vi "ISMBUS_DecodeModuleProtocol.vi"(8 "Fehler (Eingang - kein Fehler)":errorcluster, 11 "ModuleProtocolIndex":i32) -> (0 "error (Ausgang)":errorcluster caption="Fehler  (Ausgang)", 3 "ModuleProtocolString":string)   [LabVIEW 2016]
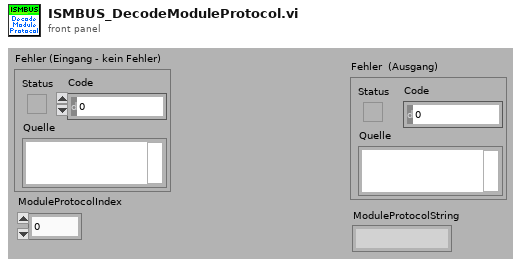
[diagram p1: front panel]
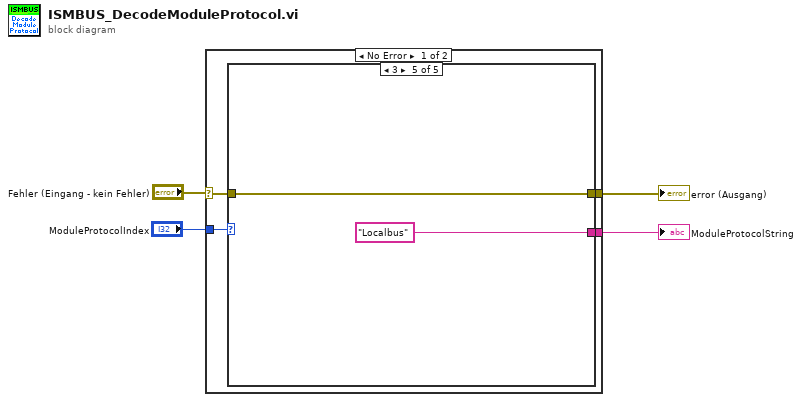
[diagram p0: block diagram]
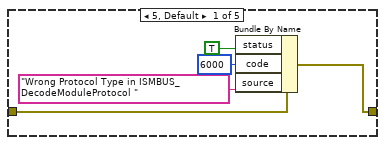
[diagram p2: hidden frame]
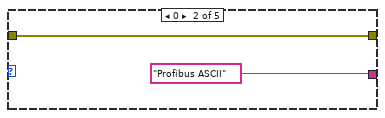
[diagram p3: hidden frame]
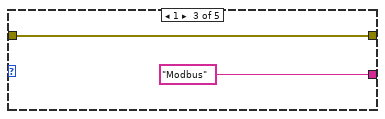
[diagram p4: hidden frame]
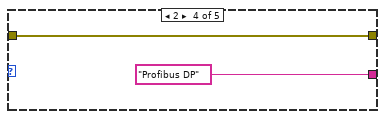
[diagram p5: hidden frame]
diagram:
  n1 = case shown="No Error" "Fehler (Eingang - kein Fehler)" {
    selector: "Fehler (Eingang - kein Fehler)" -> [w6 w22]
    tunnel: "ModuleProtocolIndex" -> [w8 _]
    tunnel: [w7 _] -> w1
    tunnel: [w5 w22] -> w2
    frame No Error {
      n2 = case shown="3" w8 {
        tunnel: [_ "Profibus ASCII" "Modbus" "Profibus DP" "Localbus"] -> w7
        tunnel: w6 -> [w12 w15 w16 w18 w20]
        tunnel: [w13 w15 w16 w18 w20] -> w5
        frame 5, Default {
          n3 = Bundle By Name(cluster=w12, "status"=TRUE, "code"=6000, "source"="Wrong Protocol Type in ISMBUS_DecodeModuleProtocol ") -> (w13:errorcluster)
        }
        frame 0 {
        }
        frame 1 {
        }
        frame 2 {
        }
        frame 3 {
        }
      }
    }
    frame Error {
    }
  }
  "error (Ausgang)" <- w2
  "ModuleProtocolString" <- w1
